vi "drivePID.vi"() -> ()   [LabVIEW 2012]
uses:
  State_Machine_Enum.ctl
  Sally_Dashboard_2013/DBNameEnum.ctl
  RefnameEnum.ctl
  Robot Global Data.vi
  <vilib>/Rock Robotics/WPI/RobotDrive/WPI_RobotDriveGetSetRefNum.vi
panel:
  out "Loop Difference":u32
  in  "RPMRight":dbl(slide)=50.0 min=0.0 max=75.0 step=1.0 scale=0.0..75.0
  in  "RPMLeft":dbl(slide)=50.0 min=0.0 max=75.0 step=1.0 scale=0.0..75.0
  in  "output range RIGHT":cluster{"output high":dbl, "output low":dbl}={"output high"=1.0, "output low"=-1.0} {"output low" min=-1.0 max=1.0 step=0.1 format="%.2f"; "output high" min=-1.0 max=1.0 step=0.1 format="%.2f"}
  in  "output range LEFT":cluster{"output high":dbl, "output low":dbl}={"output high"=1.0, "output low"=-1.0} {"output low" min=-1.0 max=1.0 step=0.1 format="%.2f"; "output high" min=-1.0 max=1.0 step=0.1 format="%.2f"}
  in  "PID RIGHT":T1={"proportional gain (Kc)"=0.015, "integral time (Ti, min)"=0.001, "derivative time (Td, min)"=0.0} {"derivative time (Td, min)" format="%.3f"; "integral time (Ti, min)" format="%.3f"; "proportional gain (Kc)" format="%.3f"}
  in  "PID LEFT":T1={"proportional gain (Kc)"=0.015, "integral time (Ti, min)"=0.001, "derivative time (Td, min)"=0.0} {"derivative time (Td, min)" format="%.3f"; "integral time (Ti, min)" format="%.3f"; "proportional gain (Kc)" format="%.3f"}
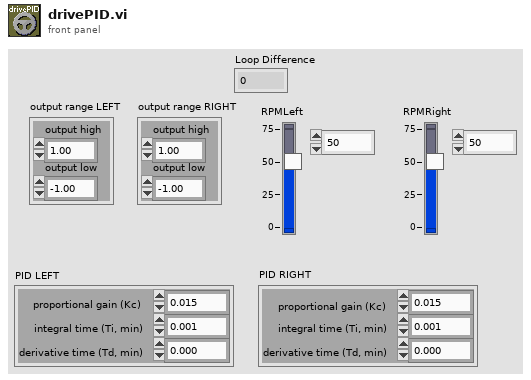
[diagram p1: front panel]
types:
  T1 = cluster{"proportional gain (Kc)":dbl, "integral time (Ti, min)":dbl, "derivative time (Td, min)":dbl}
  T2 = typedef "State_Machine_Enum.ctl" = enum16{"Idle", "Start", "Do", "Stop", "Init"}
  T3 = typedef "DBNameEnum.ctl" = enum16{"AutoEnum", "DriveLoopTime", "DriveAlignLS", "ClimbLS", "LauncherAngleMatches", "FrameworkVersion", "sLauncherAngle", "LauncherTargetAngle", "sLauncherRPM", "LauncherTargetRPM", "sDriveDistance", "LauncherMotorValue", "PullbackTol", "FireTol", "LauncherRPMTol", "LauncherAngleTol", "BackRight", "CloseLeft", "BehindPyramid", "Disabled", "CloseRight", "BackLeft", "InitialWait", "WaitBetweenLaunch", "AngleCluster", "RPMCluster", "UseAngleEncoder", "UseLauncherEncoder", "UseLauncherPID"}
  T4 = typedef "RefnameEnum.ctl" = enum16{"FireLauncher", "Climber", "Shield", "TankDrive", "DriveEncoderL", "DriveEncoderR", "LauncherMotorRPM", "LauncherEncoderAnalog", "LauncherEncoderRPM", "ShooterLS", "DriveAlignLS", "ClimbingLS", "LauncherEncoderAngle", "LauncherMotorAngle", "Gamepad1", "Gamepad2", "Compressor"}
  T5 = typedef "LoopDisable.ctl" = cluster{"Climb.vi":bool, "LauncherAngle.vi":bool, "Launcher.vi":bool, "ArmControl.vi":bool, "WinchMotor.vi":bool, "ReadDriveEncoder.vi":bool}
  T6 = typedef "WPI_DigitalInputDevRef.ctl" = cluster{"DevStatus":errorcluster, "DIO Channel":T7, "Digital Module":T8}
  T7 = typedef "FPGA_DIOChannel.ctl" = enum8{"DIO 1", "DIO 2", "DIO 3", "DIO 4", "DIO 5", "DIO 6", "DIO 7", "DIO 8", "DIO 9", "DIO 10", "DIO 11", "DIO 12", "DIO 13", "DIO 14", "Invalid"}
  T8 = typedef "FPGA_TypedefDigitalModule.ctl" = enum16{"Digital Module 1", "Digital Module 2"}
  T9 = typedef "WPI_RobotDriveDevRef.ctl" = cluster{"DevStatus":errorcluster, "Motors[]":T10[], "Square Inputs":bool, "Max Output":dbl, "Isochronous":bool}
  T10 = typedef "WPI_MotorControlDeviceRef.ctl" = cluster{"DeviceStatus":errorcluster, "Type":enum16{"PWM", "CAN"}, "PWM":cluster{"Digital Module":T8, "PWM Channel":T11, "DeadBand":T12}, "CAN":cluster{"Device Number":u8, "Control Mode":T13, "Semaphore":T14, "Max Vout":dbl}, "Invert":bool, "TransformRef":T15, "InvTransformRef":T15}
  T11 = typedef "FPGA_DIOPWMChannel.ctl" = enum8{"PWM 1", "PWM 2", "PWM 3", "PWM 4", "PWM 5", "PWM 6", "PWM 7", "PWM 8", "PWM 9", "PWM 10", "Invalid"}
  T12 = typedef "WPI_PWMDeadband.ctl" = cluster{"Name":string, "maxPositivePwm":i32, "minPositivePwm":i32, "centerPwm":i32, "maxNegativePwm":i32, "minNegativePwm":i32, "angularRange":u16}
  T13 = typedef "WPI_CANJaguar_ControlMode.ctl" = enum8{"Percent VBus", "Current", "Speed", "Position", "Voltage"}
  T14 = typedef "Semaphore RefNum" = refnum<k1>
  T15 = typedef "WPI_PWMTransform_ConPane.ctl" = refnum<vi>
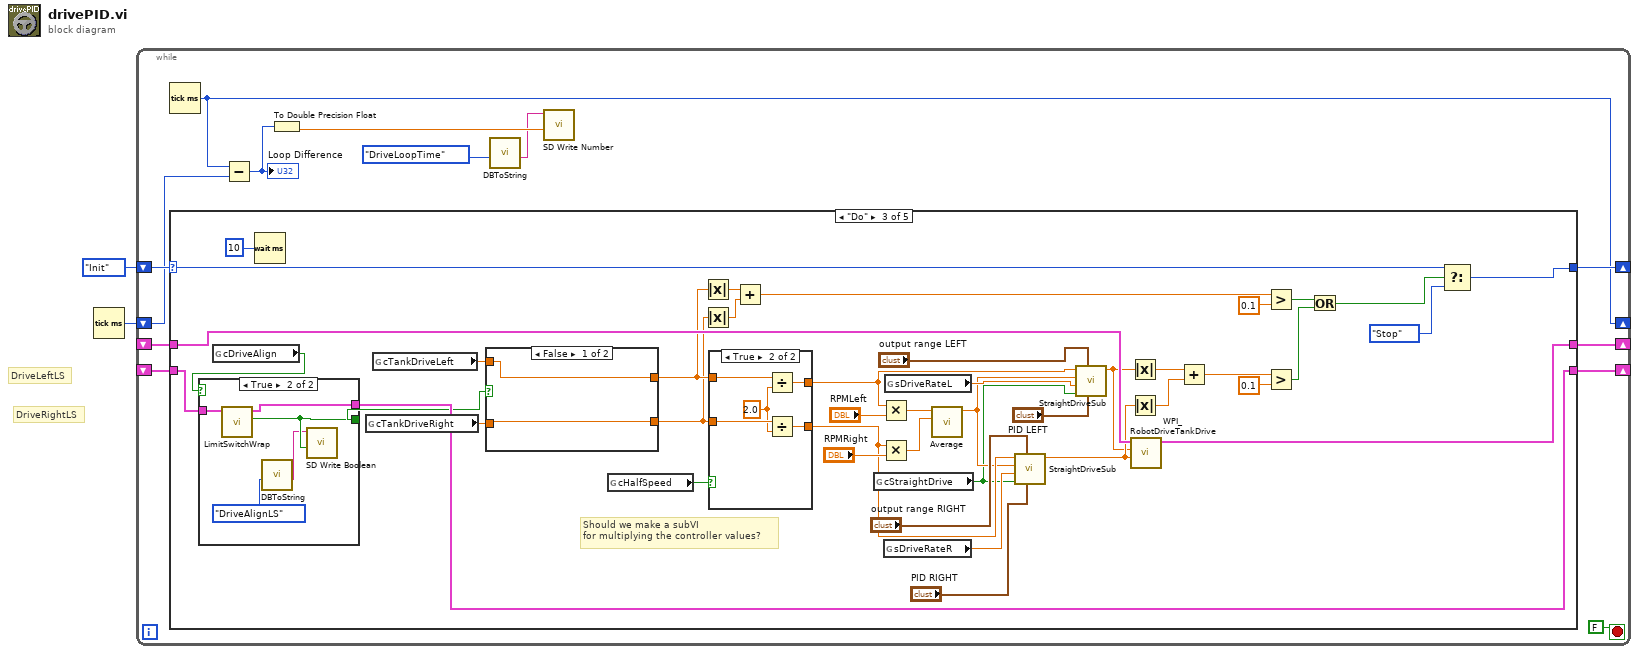
[diagram p0: block diagram]
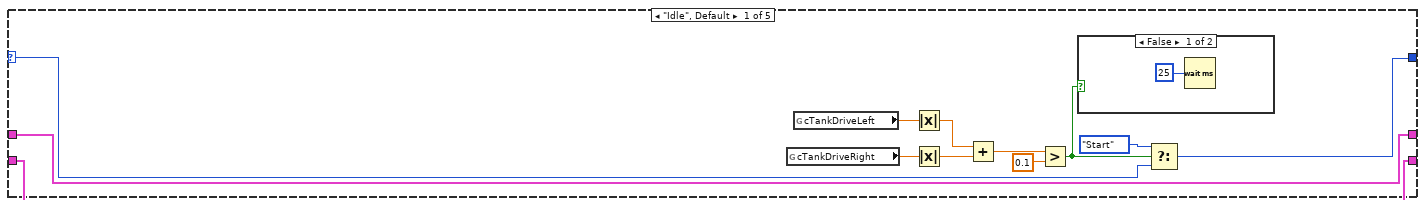
[diagram p2: hidden frame]
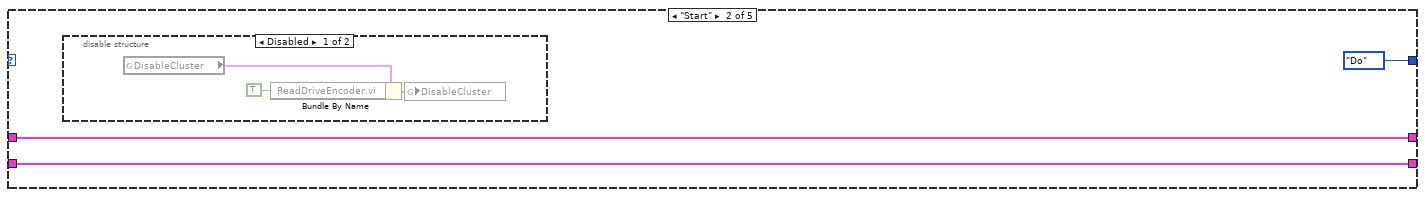
[diagram p4: hidden frame]
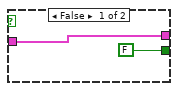
[diagram p6: hidden frame]
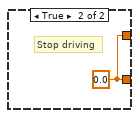
[diagram p7: hidden frame]
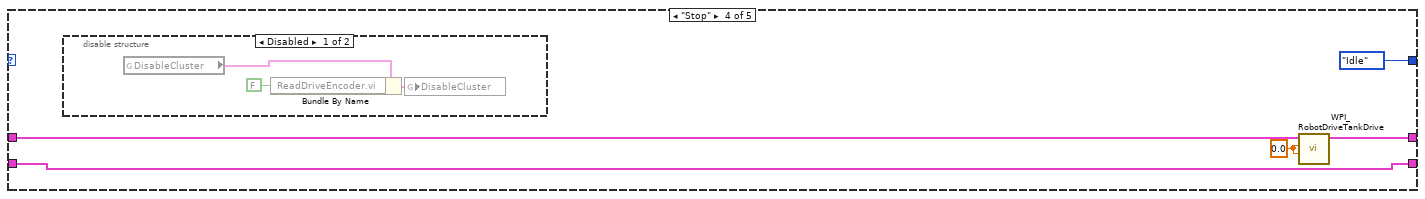
[diagram p9: hidden frame]
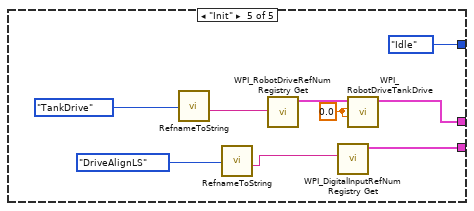
[diagram p11: hidden frame]
diagram:
  # "DriveRightLS"
  # "DriveLeftLS"
  n1 = Tick Count (ms)() -> (millisecond timer value=w1:u32)
  n2 = while {
    shift-right: [w13] -> _
    shift-left: State_Machine_Enum."Init" ("State") -> [w12]
    shift-right: [w14] -> _
    shift-left: _ -> [w15]
    shift-right: [w8] -> _
    shift-left: w1 -> [w7]
    shift-right: [w6] -> _
    shift-left: _ -> [w5]
    stop <- FALSE stop-if-true
    n3 = Tick Count (ms)() -> (millisecond timer value=w8:u32)
    n4 = case shown="\"Do\"" w12 {
      selector: w12 -> [w18 _ w71 _ _]
      tunnel: w15 -> [w17 w31 w73 w98 _]
      tunnel: [w17 w31 w62 w97 w108] -> w14
      tunnel: [w19 State_Machine_Enum."Do" ("State") w72 State_Machine_Enum."Idle" ("State") State_Machine_Enum."Idle" ("State")] -> w13
      tunnel: [w16 w29 w36 w94 w106] -> w6
      tunnel: w5 -> [w16 w29 w37 w94 _]
      frame "Idle", Default {
        n5 = global read "Robot Global Data.vi" "cTankDriveRight"() -> (w22:dbl)
        n6 = global read "Robot Global Data.vi" "cTankDriveLeft"() -> (w23:dbl)
        n7 = Absolute Value(x=w23) -> (abs(x)=w27:dbl)
        n8 = Absolute Value(x=w22) -> (abs(x)=w26:dbl)
        n9 = Add(x=w27, y=w26) -> (x+y=w25:dbl)
        n10 = Greater?(x=w25, y=0.1) -> (0:w20:bool)
        n11 = case shown="False" w20 {
          frame False {
            n12 = Wait (ms)(milliseconds to wait=u32 25) -> ()  [unwired: 1 out]
          }
          frame True {
          }
        }
        n13 = Select(t=State_Machine_Enum."Start" ("State"), s=w20, f=w18) -> (s? t:f=w19:T2)
      }
      frame "Start" {
        n14 = disable-structure shown="Disabled" {
          frame Disabled {
            n15 = global read "Robot Global Data.vi" "DisableCluster"() -> (w34:T5)
            n16 = Bundle By Name(cluster=w34, "ReadDriveEncoder.vi"=TRUE) -> (w32:T5)
            n17 = global write "Robot Global Data.vi" "DisableCluster"(w32) -> ()
          }
          frame Enabled {
          }
        }
      }
      frame "Do" {
        # "Should we make a subVI\nfor multiplying the controller values?"
        n18 = global read "Robot Global Data.vi" "cDriveAlign"() -> (w38:bool)
        n19 = case shown="True" w38 {
          tunnel: w37 -> [w78 w83]
          tunnel: [w78 w82] -> w36
          tunnel: [FALSE ("Triggered") w81] -> w35
          frame False {
          }
          frame True {
            n20 = call "LimitSwitchWrap.vi"("DigitalInputDevRef"=w83) -> ("Triggered"=w81:bool, "DigitalInputDevRef 2"=w82:T6)  [unwired: 9 in]
            n21 = call "DBToString.vi"("Enum"=DBNameEnum."DriveAlignLS") -> ("Refname"=w79:string)  [unwired: 9 in]
            n22 = call <vilib>:"SD Write Boolean.vi"("Boolean"=w81, "Name"=w79) -> ()  [unwired: 8 in, 2 out]
          }
        }
        n23 = Wait (ms)(milliseconds to wait=u32 10) -> ()  [unwired: 1 out]
        n24 = global read "Robot Global Data.vi" "cTankDriveRight"() -> (w39:dbl)
        n25 = global read "Robot Global Data.vi" "cTankDriveLeft"() -> (w40:dbl)
        n26 = case shown="False" w35 {
          tunnel: [w85 w86] -> w45
          tunnel: [w84 w86] -> w44
          tunnel: w40 -> [w85 _]
          tunnel: w39 -> [w84 _]
          frame False {
          }
          frame True {
            w86 = 0.0
            # "Stop driving"
          }
        }
        n27 = global read "Robot Global Data.vi" "cHalfSpeed"() -> (w41:bool)
        n28 = Absolute Value(x=w45) -> (abs(x)=w47:dbl)
        n29 = Absolute Value(x=w44) -> (abs(x)=w46:dbl)
        n30 = case shown="True" w41 {
          tunnel: w44 -> [w87 w92]
          tunnel: w45 -> [w88 w93]
          tunnel: [w88 w89] -> w53
          tunnel: [w87 w90] -> w60
          frame False {
          }
          frame True {
            w91 = 2.0
            n31 = Divide(x=w93, y=w91) -> (x/y=w89:dbl)
            n32 = Divide(x=w92, y=w91) -> (x/y=w90:dbl)
          }
        }
        n33 = Add(x=w47, y=w46) -> (x+y=w48:dbl)
        n34 = global read "Robot Global Data.vi" "cStraightDrive"() -> (w54:bool)
        n35 = Multiply(x=w53, y="RPMLeft") -> (x*y=w76:dbl)
        n36 = Multiply(x=w60, y="RPMRight") -> (x*y=w75:dbl)
        n37 = global read "Robot Global Data.vi" "sDriveRateR"() -> (w61:dbl)
        n38 = global read "Robot Global Data.vi" "sDriveRateL"() -> (w56:dbl)
        n39 = call "Average.vi"("y"=w75, "x"=w76) -> ("x/y"=w55:dbl)  [unwired: 9 in]
        n40 = call "StraightDriveSub.vi"("PID Constants"="PID RIGHT", "output range"="output range RIGHT", "StraightDriveEngage?"=w54, "sDriveRate"=w61, "Average Controller Value"=w55, "Controller Value"=w60) -> ("Motor Value"=w59:dbl)  [unwired: 5 in]
        n41 = call "StraightDriveSub.vi"("PID Constants"="PID LEFT", "output range"="output range LEFT", "StraightDriveEngage?"=w54, "sDriveRate"=w56, "Average Controller Value"=w55, "Controller Value"=w53) -> ("Motor Value"=w52:dbl)  [unwired: 5 in]
        n42 = Absolute Value(x=w52) -> (abs(x)=w65:dbl)
        n43 = Absolute Value(x=w59) -> (abs(x)=w64:dbl)
        n44 = call <vilib>:"WPI_RobotDriveTankDrive.vi"("Right axis value"=w59, "Left axis value"=w52, "RobotDriveDevRef"=w73) -> ("RobotDriveDevRef"=w62:T9)  [unwired: 6 in, 2 out]
        n45 = Add(x=w65, y=w64) -> (x+y=w66:dbl)
        n46 = Greater?(x=w48, y=0.1) -> (0:w42:bool)
        n47 = Greater?(x=w66, y=0.1) -> (0:w43:bool)
        n48 = Or(x=w42, y=w43) -> (x .or. y?=w63:bool)
        n49 = Select(t=w71, s=w63, f=State_Machine_Enum."Stop") -> (s? t:f=w72:T2)
      }
      frame "Stop" {
        w96 = 0.0 ("Right axis value")
        n50 = disable-structure shown="Disabled" {
          frame Disabled {
            n51 = global read "Robot Global Data.vi" "DisableCluster"() -> (w101:T5)
            n52 = Bundle By Name(cluster=w101, "ReadDriveEncoder.vi"=FALSE) -> (w99:T5)
            n53 = global write "Robot Global Data.vi" "DisableCluster"(w99) -> ()
          }
          frame Enabled {
          }
        }
        n54 = call <vilib>:"WPI_RobotDriveTankDrive.vi"("Right axis value"=w96, "Left axis value"=w96, "RobotDriveDevRef"=w98) -> ("RobotDriveDevRef"=w97:T9)  [unwired: 6 in, 2 out]
      }
      frame "Init" {
        w109 = 0.0 ("Left axis value")
        n55 = call "RefnameToString.vi"("Enum"=RefnameEnum."TankDrive") -> ("Refname"=w104:string)  [unwired: 10 in]
        n56 = call "RefnameToString.vi"("Enum"=RefnameEnum."DriveAlignLS") -> ("Refname"=w102:string)  [unwired: 10 in]
        n57 = call <vilib>:"WPI_RobotDriveRefNum Registry Get.vi"("refnum name"=w104) -> ("RobotDriveDevRef"=w110:T9)  [unwired: 9 in, 1 out]
        n58 = call <vilib>:"WPI_DigitalInputRefNum Registry Get.vi"("refnum name"=w102) -> ("DigitalInputDevRef"=w106:T6)  [unwired: 9 in, 1 out]
        n59 = call <vilib>:"WPI_RobotDriveTankDrive.vi"("Right axis value"=w109, "Left axis value"=w109, "RobotDriveDevRef"=w110) -> ("RobotDriveDevRef"=w108:T9)  [unwired: 6 in, 2 out]
      }
    }
    n60 = Subtract(x=w8, y=w7) -> (x-y=w10:u32)
    "Loop Difference" <- w10
    n61 = To Double Precision Float(number=w10) -> (double precision float=w9:dbl)
    n62 = call "DBToString.vi"("Enum"=DBNameEnum."DriveLoopTime") -> ("Refname"=w3:string)  [unwired: 9 in]
    n63 = call <vilib>:"SD Write Number.vi"("Numeric"=w9, "Name"=w3) -> ()  [unwired: 8 in, 2 out]
  }
